vi "扫描.vi"(5 "坐标轴映射":T1, 6 "测试数据":dbl[][](array[numeric]), 7 "XY图":refnum<vi>, 8 "曲线设置":T2={"X轴数据选择"=enum."设置电压", "Y轴组"=[]}, 10 "错误输入（无错误）":errorcluster, 11 "保留数量":i32) -> (2 "错误输出":errorcluster, 3 "突变电压":dbl)   [LabVIEW 2021]
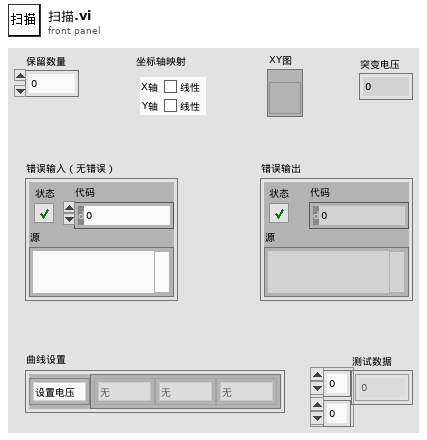
[diagram p1: front panel]
types:
  T1 = typedef "坐标轴映射.ctl" = cluster{"X轴":bool, "Y轴":bool}
  T2 = typedef "曲线设置.ctl" = cluster{"X轴数据选择":enum16{"时间", "设置电压", "读取电流", "读取电压"}, "Y轴组":enum16{"时间", "设置电压", "读取电流", "读取电压", "无"}[]}
  T3 = cluster{"Name":string, "Color":u32, "Style":u8, "Point Style":u8, "Name Visible":bool, "Allow Drag":bool, "Cursor Mode":u32, "Plot":i32, "Index":i32, "Position":cluster{"X":dbl, "Y":dbl}, "X Scale":u32, "Y Scale":u32, "Watch Plots":i32[], "Watch All Plots":bool, "Plot Area":i32, "Label Offset":cluster{"X":i32, "Y":i32}}
  T4 = cluster{"Name":string, "Color":u32, "Style":u8, "Point Style":u8, "Name Visible":bool, "Allow Drag":bool, "Cursor Mode":u32, "Plot":i32, "Index":i32, "Position":cluster{"X":dbl, "Y":dbl}, "X Scale":u32, "Y Scale":u32, "Watch Plots":i32[], "Watch All Plots":bool, "Plot Area":i32, "Label Offset":cluster{"X":i32, "Y":i32}}[]
  T5 = typedef "曲线属性.ctl" = cluster{"曲线名":string, "曲线颜色":u32}
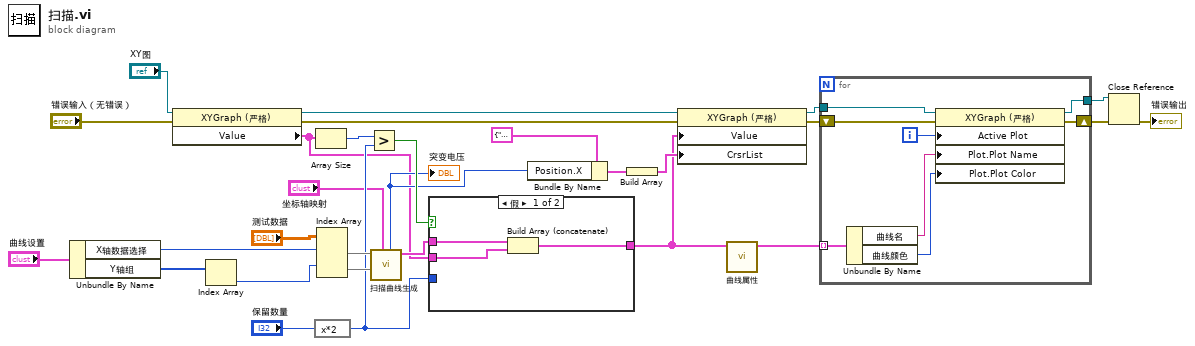
[diagram p0: block diagram]
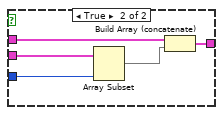
[diagram p2: hidden frame]
diagram:
  n1 = Unbundle By Name("曲线设置") -> ("X轴数据选择"=w28:enum16{"时间", "设置电压", "读取电流", "读取电压"}, "Y轴组"=w27:enum16{"时间", "设置电压", "读取电流", "读取电压", "无"}[])
  n2 = property class="XYGraph (严格)"(reference="XY图", error in="错误输入（无错误）") -> (reference out=w21:refnum<vi>, error out=w20:errorcluster, "Value"=w3:cluster{"测试数据":dbl[], "测试数据":dbl[]}[])
  n3 = Index Array(array=w27) -> (element=w29:enum16{"时间", "设置电压", "读取电流", "读取电压", "无"})  [unwired: 1 in]
  n4 = expression code="x*2"("保留数量") -> (w5:i32)
  n5 = Array Size(array=w3) -> (size(s)=w13:i32)
  n6 = Index Array(array="测试数据", index (row) #1=w28, index (row) #2=w29) -> (element #1=w9:dbl[], element #2=w26:dbl[])  [unwired: 2 in]
  n7 = Greater?(x=w13, y=w5) -> (0:w14:bool)
  n8 = call "扫描曲线生成.vi"("坐标轴映射"="坐标轴映射", "Y"=w26, "X"=w9) -> ("曲线"=w7:cluster{dbl[], dbl[]}[], "突变电压"=w8:i32)  [unwired: 7 in]
  "突变电压" <- w8
  n9 = case shown="假" w14 {
    tunnel: w3 -> [w31 w37]
    tunnel: [w32 w36] -> w2
    tunnel: w5 -> [_ w33]
    tunnel: w7 -> [w30 w34]
    frame False {
      n10 = Build Array (concatenate)(w30, w31) -> (w32:cluster{"测试数据":dbl[], "测试数据":dbl[]}[])
    }
    frame True {
      n11 = Array Subset(array=w37, length=w33) -> (w35:cluster{"测试数据":dbl[], "测试数据":dbl[]}[])  [unwired: 1 in]
      n12 = Build Array (concatenate)(w34, w35) -> (w36:cluster{"测试数据":dbl[], "测试数据":dbl[]}[])
    }
  }
  n13 = Bundle By Name(cluster=T3 {"Name"="游标", "Color"=16776960, "Style"=2, "Point Style"=13, "Name Visible"=FALSE, "Allow Drag"=TRUE, "Cursor Mode"=2, "Plot"=-1, "Index"=0, "Position"={"X"=0.0, "Y"=0.0}, "X Scale"=0, "Y Scale"=0, "Watch Plots"=[], "Watch All Plots"=TRUE, "Plot Area"=0, "Label Offset"={"X"=0, "Y"=0}}, "Position.X"=w8) -> (w10:T3)
  n14 = Build Array(w10) -> (w4:T4)
  n15 = property class="XYGraph (严格)"(reference=w21, error in=w20, "Value"=w2, "CrsrList"=w4) -> (reference out=w19:refnum<vi>, error out=w18:errorcluster)
  n16 = call "曲线属性.vi"("曲线"=w2) -> ("曲线属性"=w12:T5[])  [unwired: 10 in]
  n17 = for {
    shift-right: [w44] -> w17
    shift-left: w18 -> [w45]
    tunnel: w12 -> [w38] mode=indexing
    tunnel: w19 -> [w43]
    tunnel: [w42] -> w16
    i -> [w41]
    n18 = Unbundle By Name(w38) -> ("曲线名"=w40:string, "曲线颜色"=w39:u32)
    n19 = property on="属性节点" class="XYGraph (严格)"(reference=w43, error in=w45, "Active Plot"=w41, "Plot.Plot Name"=w40, "Plot.Plot Color"=w39) -> (reference out=w42:refnum<vi>, error out=w44:errorcluster)
  }
  n20 = Close Reference(reference=w16, error in (no error)=w17) -> (error out=→"错误输出":errorcluster)
